vi "Contour Line_Prepare XY Inputs.vi"(9 "Z In":dbl[][](array[numeric]), 10 "Y In":dbl[](array[numeric]), 11 "X In":dbl[](array[numeric])) -> (0 "error":i32, 2 "Y Out":dbl[](array[numeric]), 3 "X Out":dbl[](array[numeric]))   [LabVIEW 2017, in "NI_AAL_Geometry.lvlib"]
uses:
  <vilib>/Analysis/NI_AAL_Geometry.lvlib
  <vilib>/Analysis/1siggen.llb/Ramp Pattern by Samples.vi
  <vilib>/Analysis/NI_AALBase.lvlib
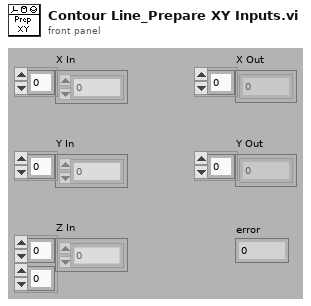
[diagram p1: front panel]
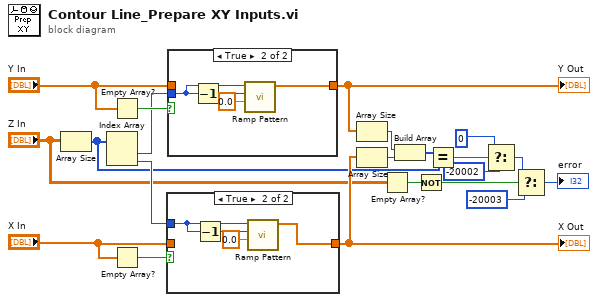
[diagram p0: block diagram]
diagram:
  n1 = Array Size(array="Z In") -> (size(s)=w6:i32[])
  n2 = Index Array(array=w6) -> (element #1=w19:i32, element #2=w18:i32)  [unwired: 2 in]
  n3 = Empty Array?(array="Y In") -> (empty?=w20:bool)
  n4 = Empty Array?(array="X In") -> (empty?=w21:bool)
  n5 = case shown="True" w21 {
    tunnel: w18 -> [_ w24]
    tunnel: [w22 w25] -> w13
    tunnel: "X In" -> [w22 _]
    frame False {
    }
    frame True {
      n6 = Decrement(x=w24) -> (x-1=w23:i32)
      n7 = call-poly <vilib>:"Ramp Pattern.vi"("start"=0.0, "end"=w23, "samples"=w24) -> ("Ramp Pattern"=w25:dbl[])  [unwired: 7 in, 1 out]
    }
  }
  "X Out" <- w13
  n8 = case shown="True" w20 {
    tunnel: w19 -> [_ w28]
    tunnel: [w27 w30] -> w14
    tunnel: "Y In" -> [w27 _]
    frame False {
    }
    frame True {
      n9 = Decrement(x=w28) -> (x-1=w29:i32)
      n10 = call-poly <vilib>:"Ramp Pattern.vi"("start"=0.0, "end"=w29, "samples"=w28) -> ("Ramp Pattern"=w30:dbl[])  [unwired: 7 in, 1 out]
    }
  }
  "Y Out" <- w14
  n11 = Array Size(array=w14) -> (size(s)=w12:i32)
  n12 = Array Size(array=w13) -> (size(s)=w11:i32)
  n13 = Empty Array?(array="Z In") -> (empty?=w4:bool)
  n14 = Build Array(w12, w11) -> (w15:i32[])
  n15 = Not(x=w4) -> (.not. x?=w1:bool)
  n16 = Equal?(x=w15, y=w6) -> (x = y?=w10:bool)
  n17 = Select(t=0, s=w10, f=-20002) -> (s? t:f=w3:i32)
  n18 = Select(t=w3, s=w1, f=-20003) -> (s? t:f=→"error":i32)
